vi "Sample Inputs.vi"(0 "Sampling Period (ms) (50ms)":i64=50, 1 "Num Samples  to Average (5)":i32=5) -> (6 "ADC Readings (filtered)":T1)   [LabVIEW 2017]
uses:
  <vilib>/Platform/TimedLoop/XDataNode/timing_clust.ctl
  <vilib>/Platform/TimedLoop/XDataNode/nitl_modes.ctl
  <vilib>/Platform/TimedLoop/XDataNode/wakeup.ctl
  <vilib>/myRIO/Instrument Drivers/Onboard IO/AI/typedefs/AI Reference.ctl
  <vilib>/myRIO/Common/Instrument Driver Framework/Utilities/typedefs/myRIO Generic Hardware Reference.ctl
  <vilib>/myRIO/Common/Instrument Driver Framework/Utilities/typedefs/Hardware Version Enum.ctl
  <vilib>/myRIO/Common/Instrument Driver Framework/Utilities/typedefs/myRIO v1.0 Reference.ctl
  <vilib>/myRIO/Common/Instrument Driver Framework/Utilities/typedefs/Generic FPGA Reference.ctl
  <vilib>/myRIO/Common/Instrument Driver Framework/myRIO v1.0/AI/typedefs/AI Channels List.ctl
  <vilib>/myRIO/Common/Instrument Driver Framework/myRIO v1.0/AI/typedefs/AI Channels Enum.ctl
  <vilib>/myRIO/Common/Instrument Driver Framework/Utilities/typedefs/Analog Scaling Constants List.ctl
  <vilib>/myRIO/Common/Instrument Driver Framework/Utilities/typedefs/Analog Scaling Constants.ctl
  <vilib>/userdefined/High Color/nirio_resource_hc.ctl
  <vilib>/myRIO/Common/Instrument Driver Framework/Utilities/vis/Is FPGA Ref Available.vi
  <vilib>/myRIO/Common/Instrument Driver Framework/myRIO v1.0/AI/vis/myRIO v1.1 Open AI.vi
  <vilib>/myRIO/Instrument Drivers/Onboard IO/AI/vis/Read.vi
  <vilib>/myRIO/Common/Instrument Driver Framework/Utilities/vis/Validate Channels.vi
  <vilib>/myRIO/Common/Instrument Driver Framework/myRIO v1.0/AI/vis/myRIO v1.0 Reserve AI.vi
  <vilib>/myRIO/Common/Instrument Driver Framework/myRIO v1.0/AI/vis/myRIO v1.0 Build MUX Configuration AI.vi
  <vilib>/myRIO/Common/Instrument Driver Framework/myRIO v1.0/Resource Manager/vis/myRIO v1.0 Reserve Channel List.vi
  <vilib>/myRIO/Common/Instrument Driver Framework/myRIO v1.0/Resource Manager/vis/myRIO v1.0 Reserve Channel.vi
  <vilib>/myRIO/Common/Instrument Driver Framework/myRIO v1.0/Resource Manager/vis/myRIO v1.0 Unreserve Channel.vi
  <vilib>/myRIO/Common/Instrument Driver Framework/myRIO v1.0/Resource Manager/vis/myRIO v1.0 Build Mutex Name.vi
  <vilib>/Utility/VariantDataType/GetNumericInfo.vi
  <vilib>/Utility/error.llb/Error Cluster From Error Code.vi
  <vilib>/myRIO/Common/Instrument Driver Framework/myRIO v1.0/myRIO v1.1 Open.vi
  <vilib>/myRIO/Common/Instrument Driver Framework/myRIO v1.0/AI/vis/myRIO v1.0 Get Scaling Constants AI.vi
  <vilib>/myRIO/Common/Instrument Driver Framework/Utilities/vis/IO Manager.vi
  <vilib>/myRIO/Common/Instrument Driver Framework/Utilities/vis/Configuration Manager.vi
  <vilib>/myRIO/Common/Instrument Driver Framework/myRIO v1.0/myRIO v1.0 Close.vi
  <vilib>/myRIO/Common/Instrument Driver Framework/myRIO v1.0/AI/vis/myRIO v1.0 Read AI.vi
  <vilib>/platform/TimedLoop/XDataNode/XDataNode.xnode
  <vilib>/myRIO/Express VI/Onboard IO/AI/AI Express VI.xnode
  <vilib>/myRIO/Instrument Drivers/Onboard IO/AI/vis/myRIO AI Open.xnode
  <vilib>/Platform/TimedLoop/XDataNode/XDNodeRunTimeDep.lvlib
  <vilib>/myRIO/Instrument Drivers/Onboard IO/AI/AI.lvlib
panel:
  out "Iout Voltage (A/AI2 (Pin 7))":dbl
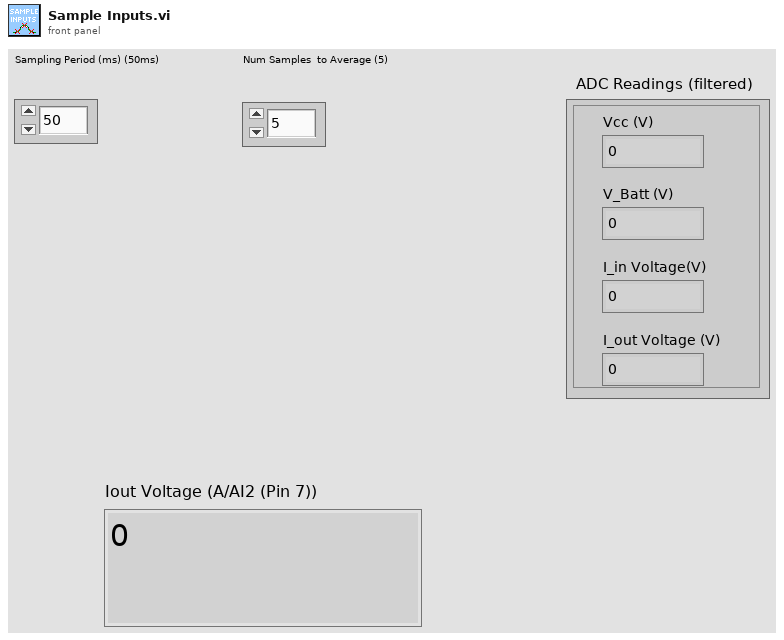
[diagram p1: front panel]
types:
  T1 = cluster{"Vcc (V)":dbl, "V_Batt (V)":dbl, "I_in Voltage(V)":dbl, "I_out Voltage (V)":dbl}
  T2 = typedef "XDNodeRunTimeDep.lvlib/timing_clust.ctl" = cluster{"Expected End [f-1]":u64, "Actual End [f-1]":u64, "Finished Late? [f-1]":bool, "Expected End [i-1]":u64, "Actual End [i-1]":u64, "Finished Late? [i-1]":bool, "Expected Start [i]":u64, "Actual Start [i]":u64, "Expected Start [f]":u64, "Actual Start [f]":u64, "Source Name":string, "Structure Name":string, "Period":i64, "Deadline":i64, "Offset":i64, "Start":i64, "Priority":i32, "Timeout":i32, "Mode":T3, "Wakeup Reason":T4, "Error":errorcluster, "Source Type":string, "Secondary Source Type":string, "Global End Time":u64, "Global Start Time":u64, "Frame Duration":u64, "Iteration Duration":u64, "Assigned CPU":i32, "I/O Scan Engine Mode":u32}
  T3 = typedef "XDNodeRunTimeDep.lvlib/nitl_modes.ctl" = enum32{"No Change", "Process missed periods, maintain original phase", "Discard missed periods, maintain original phase", "Process missed periods, ignore original phase", "Discard missed periods, ignore original phase"}
  T4 = typedef "XDNodeRunTimeDep.lvlib/wakeup.ctl" = enum32{"Normal", "Aborted", "Asynchronous wakeup", "Timing source error", "Timed loop error", "Timeout"}
  T5 = typedef "AI.lvlib/AI Reference.ctl" = cluster{"myRIO Reference":T6, "AI Channels List":T10, "AI Scaling Constants List":T12}
  T6 = typedef "myRIO Generic Hardware Reference.ctl" = cluster{"myRIO Model":T7, "myRIO Hardware Reference":T8}
  T7 = typedef "Hardware Version Enum.ctl" = enum16{"Unknown", "myRIO-1900", "myRIO-1950", "roboRIO", "NI ELVIS RIO CM"}
  T8 = typedef "myRIO v1.0 Reference.ctl" = cluster{"Generic FPGA Reference":T9, "Allow multiple opens":bool}
  T9 = typedef "Generic FPGA Reference.ctl" = refnum<k20>
  T10 = typedef "AI Channels List.ctl" = T11[]
  T11 = typedef "AI Channels Enum.ctl" = enum16{"Not Connected", "AudioIn/Left", "AudioIn/Right", "C/AI0", "C/AI1", "A/AI0", "A/AI1", "A/AI2", "A/AI3", "B/AI0", "B/AI1", "B/AI2", "B/AI3", "AI/AI0", "AI/AI1", "AI/AI2", "AI/AI3"}
  T12 = typedef "Analog Scaling Constants List.ctl" = T13[]
  T13 = typedef "Analog Scaling Constants.ctl" = cluster{"LSB Weight (Volts)":dbl, "Offset (Volts)":dbl, "Signed?":bool}
  T14 = typedef "nirio_resource_hc.ctl" = tag
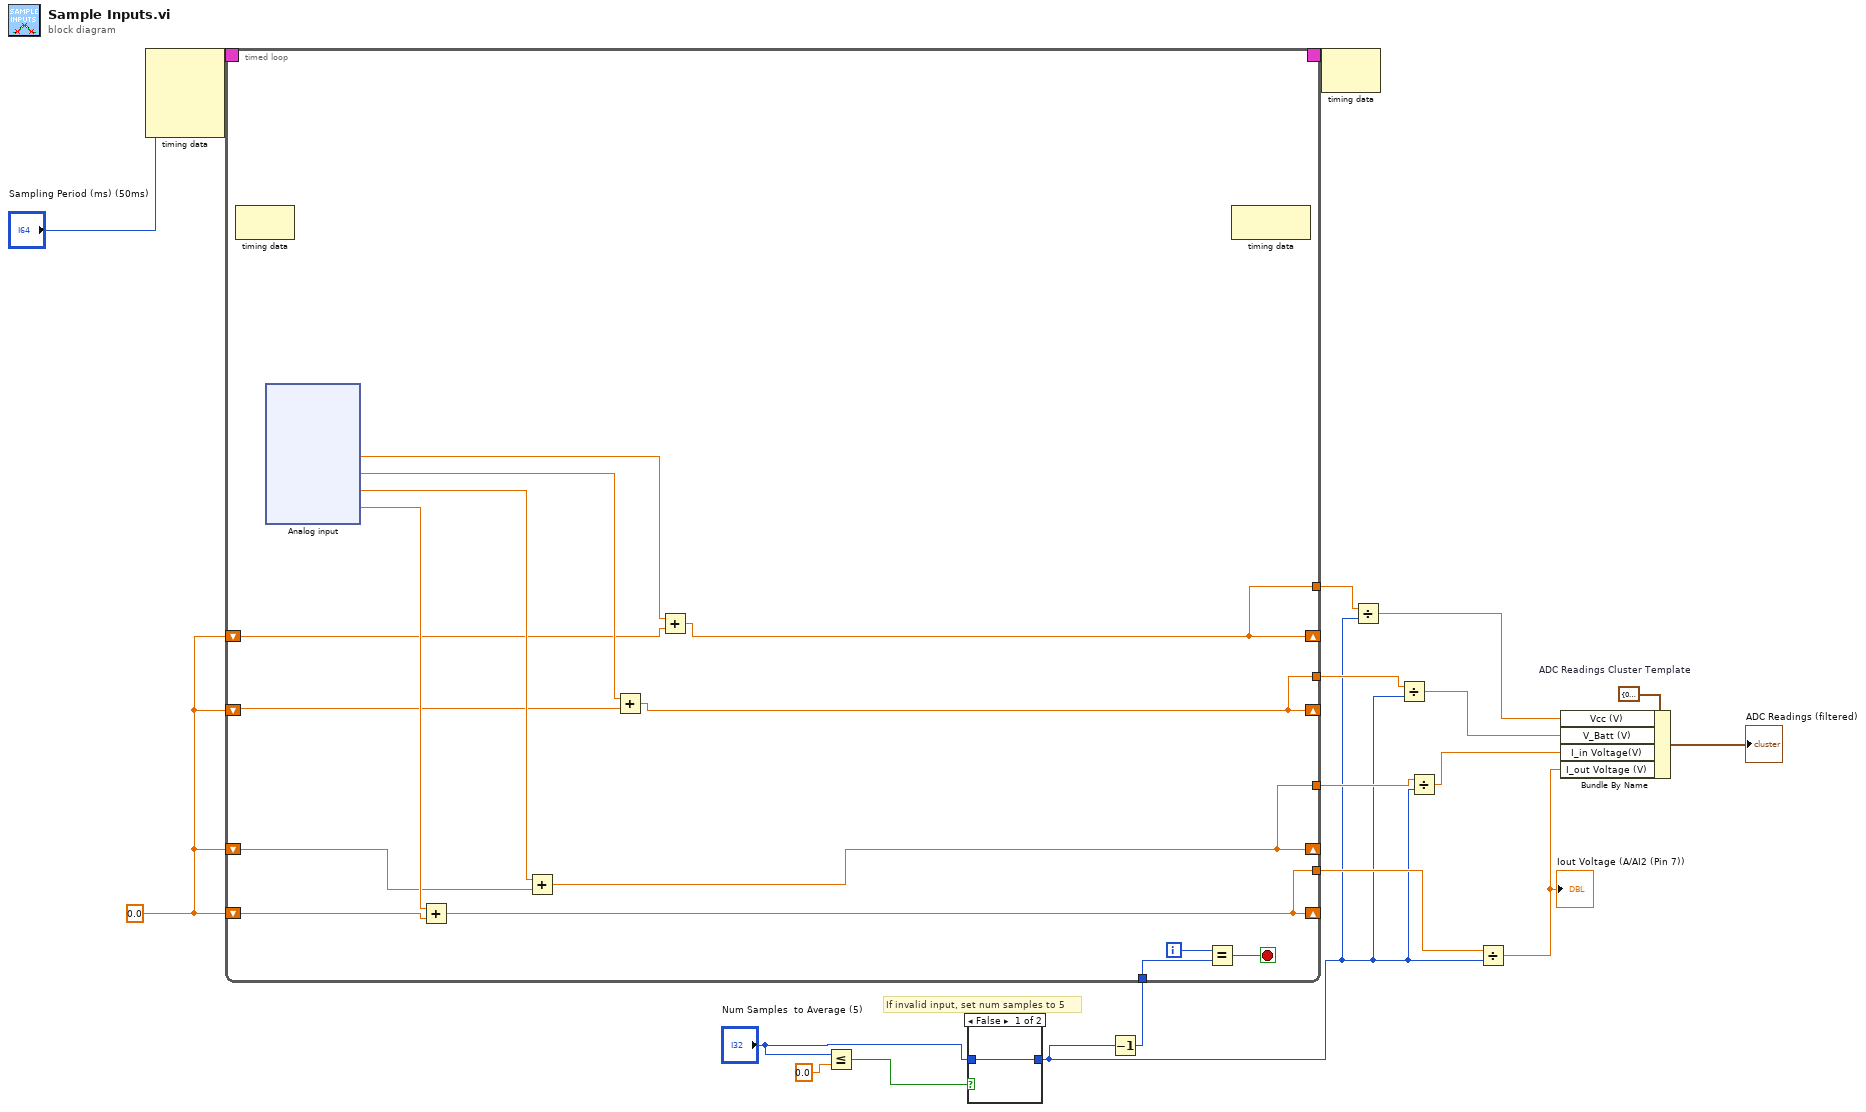
[diagram p0: block diagram]
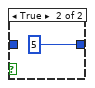
[diagram p2: hidden frame]
diagram:
  w11 = T1 {"Vcc (V)"=0.0, "V_Batt (V)"=0.0, "I_in Voltage(V)"=0.0, "I_out Voltage (V)"=0.0}  # ADC Readings Cluster Template
  w4 = 0.0
  # "If invalid input, set num samples to 5"
  n1 = node-c288("Sampling Period (ms) (50ms)") -> (w19:T2)  [unwired: 3 in]
  n2 = Less Or Equal?(x="Num Samples  to Average (5)", y=0.0) -> (x <= y?=w15:bool)
  n3 = case shown="False" w15 {
    tunnel: "Num Samples  to Average (5)" -> [w20 _]
    tunnel: [w20 5] -> w2
    frame False {
    }
    frame True {
    }
  }
  n4 = Decrement(x=w2) -> (x-1=w17:i32)
  n5 = timed-loop {
    timing: w19 -> [_]
    timing-out: [_] -> w18
    tunnel: w17 -> [w34]
    shift-right: [w32] -> _
    shift-left: w4 -> [w33]
    tunnel: [w32] -> w12
    shift-right: [w28] -> _
    shift-left: w4 -> [w30]
    tunnel: [w28] -> w9
    shift-right: [w25] -> _
    shift-left: w4 -> [w27]
    tunnel: [w25] -> w6
    shift-right: [w22] -> _
    shift-left: w4 -> [w24]
    tunnel: [w22] -> w3
    i -> [w36]
    stop <- w35 stop-if-true
    n6 = node-c288() -> ()  [unwired: 1 in, 1 out]
    n7 = xnode "Analog input"() -> ("Vcc (A/AI0 (Pin 3))"=w23:dbl, "Batt+ (A/AI1 (Pin 5))"=w26:dbl, "Iin Voltage (A/AI2 (Pin 7))"=w29:dbl, "Iout Voltage (A/AI3 (Pin 9))"=w31:dbl)  [unwired: 1 in, 1 out]
    n8 = Add(x=w31, y=w33) -> (x+y=w32:dbl)
    n9 = Add(x=w29, y=w30) -> (x+y=w28:dbl)
    n10 = Add(x=w26, y=w27) -> (x+y=w25:dbl)
    n11 = Add(x=w23, y=w24) -> (x+y=w22:dbl)
    n12 = Equal?(x=w36, y=w34) -> (x = y?=w35:bool)
    n13 = node-c288() -> ()  [unwired: 1 in, 1 out]
  }
  n14 = node-c288(w18) -> ()  [unwired: 1 out]
  n15 = Divide(x=w3, y=w2) -> (x/y=w1:dbl)
  n16 = Divide(x=w6, y=w2) -> (x/y=w5:dbl)
  n17 = Divide(x=w9, y=w2) -> (x/y=w7:dbl)
  n18 = Divide(x=w12, y=w2) -> (x/y=w8:dbl)
  "Iout Voltage (A/AI2 (Pin 7))" <- w8
  n19 = Bundle By Name(cluster=w11, "Vcc (V)"=w1, "V_Batt (V)"=w5, "I_in Voltage(V)"=w7, "I_out Voltage (V)"=w8) -> (→"ADC Readings (filtered)":T1)
